vi "sample_calibration_find_roi_centroids.vi"(7 "ROI":T1, 8 "Error In":errorcluster, 11 "Image":T2(plugin-control)) -> (0 "Error Out":errorcluster, 3 "centroids":sgl[][](array[numeric]))   [LabVIEW 2019]
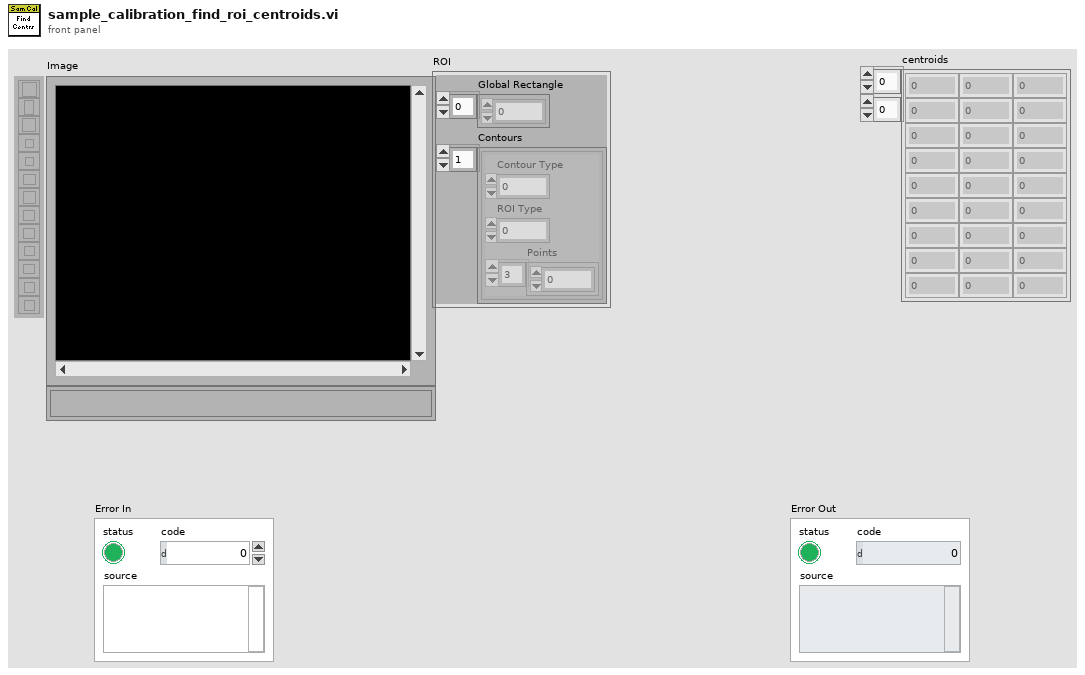
[diagram p1: front panel]
types:
  T1 = cluster{"Global Rectangle":i32[], "Contours":cluster{"Contour Type":u32, "ROI Type":u32, "Points":i32[]}[]}
  T2 = typedef "IMAQ Image.ctl" = refnum<image>
  T3 = typedef "ROI Descriptor" = cluster{"Global Rectangle":i32[], "Contours":cluster{"ID":enum32{"External", "Internal"}, "Type":u32, "Coordinates":i32[]}[]}
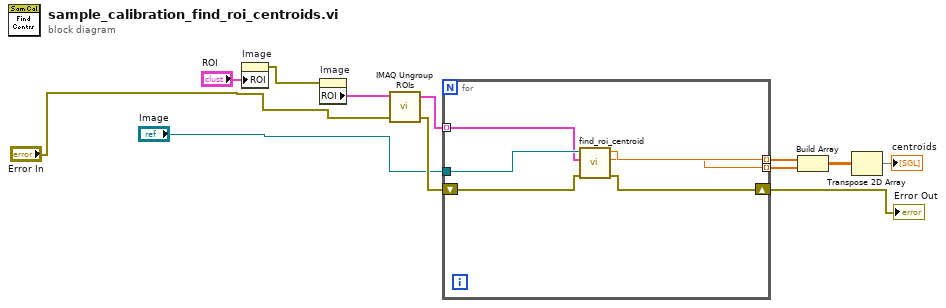
[diagram p0: block diagram]
diagram:
  n1 = property on="Image" class="ImageControl"("ROI"="ROI") -> (error out=w9:errorcluster)  [unwired: 2 in, 1 out]
  n2 = property on="Image" class="ImageControl"(error in=w9) -> ("ROI"=w12:T1)  [unwired: 1 in, 2 out]
  n3 = call "IMAQ Ungroup ROIs"("error in (no error)"="Error In", "ROI Descriptor"=w12) -> ("error out"=w11:errorcluster, "ROI Descriptors out"=w7:T3[])  [unwired: 2 in]
  n4 = for {
    tunnel: w7 -> [w15] mode=indexing
    tunnel: "Image" -> [w16]
    shift-right: [w17] -> w10
    shift-left: w11 -> [w18]
    tunnel: [w14] -> w4 mode=indexing
    tunnel: [w13] -> w3 mode=indexing
    n5 = call "find_roi_centroid.vi"("Error In"=w18, "ROI Descriptor"=w15, "Image Src"=w16) -> ("error out"=w17:errorcluster, "Y Centroid"=w13:sgl, "X Centroid"=w14:sgl)  [unwired: 6 in]
  }
  "Error Out" <- w10
  n6 = Build Array(w4, w3) -> (w6:sgl[][])
  n7 = Transpose 2D Array(2D array=w6) -> (transposed array=→"centroids":sgl[][])
